vi "To Serial Form.vi"(6 "Serial Version":T1, 10 "Serializer in":refnum<class "Serializer.lvclass">, 11 "PAS Data in":refnum<class "PAS Data.lvclass">) -> (0 "error out":errorcluster, 2 "Serializer out":refnum<class "Serializer.lvclass">, 3 "PAS Data out":refnum<class "PAS Data.lvclass">)   [LabVIEW 2014, in "PAS Data.lvclass"]
uses:
  PAS Data.lvclass
  <vilib>/NI/AQ Character Lineator/Serializer/Serializer.lvclass
  <vilib>/NI/AQ Character Lineator/Serialization Common/Serial Version.ctl
  PAS Data.lvclass/PAS Data.ctl
  Cell/PAS Cell Data.lvclass
  <vilib>/NI/AQ Character Lineator/Serializable/Insert Boolean.vi
  <vilib>/NI/AQ Character Lineator/Serializer/Insert Boolean.vi
  <vilib>/NI/AQ Character Lineator/Serializer/Read Include Default Values.vi
  Data/Data.lvclass
  <vilib>/NI/AQ Character Lineator/Serializable/Serializable.lvclass
  <vilib>/NI/AQ Character Lineator/Serialization Common/Serialization Common.lvlib
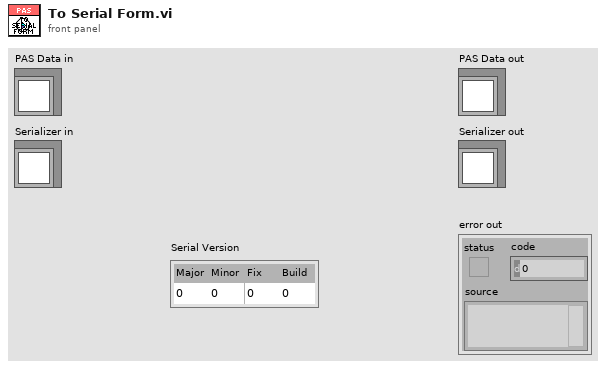
[diagram p1: front panel]
types:
  T1 = typedef "Serialization Common.lvlib/Serial Version.ctl" = cluster{"Major":u16, "Minor":u16, "Fix":u16, "Build":u16}
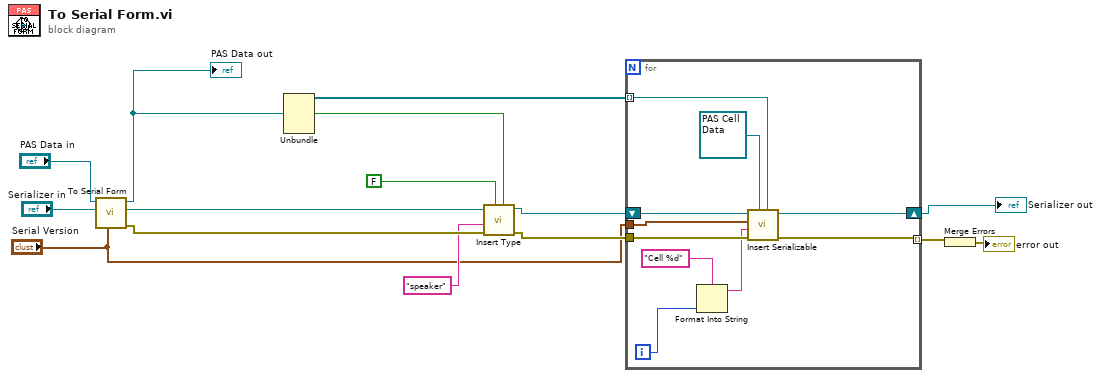
[diagram p0: block diagram]
diagram:
  n1 = call-parent "To Serial Form.vi"("Serial Version"="Serial Version", "Serializer in"="Serializer in", "Data in"="PAS Data in") -> ("error out"=w11:errorcluster, "Serializer out"=w12:refnum<class "Serializer.lvclass">, "Data out"=w13:refnum<class "PAS Data.lvclass">)  [unwired: 6 in]
  "PAS Data out" <- w13
  n2 = Unbundle(w13) -> (w7:refnum<class "PAS Cell Data.lvclass">[], w10:bool)  [unwired: 3 out]
  n3 = call-poly <vilib>:"Insert Type.vi"("Boolean"=w10, "Default Value"=FALSE, "error in (no error)"=w11, "Name"="speaker", "Serializer in"=w12) -> ("error out"=w5:errorcluster, "Serializer out"=w6:refnum<class "Serializer.lvclass">)  [unwired: 5 in]
  n4 = for {
    tunnel: w7 -> [w25] mode=indexing
    shift-right: [w22] -> w3
    shift-left: w6 -> [w23]
    tunnel: w5 -> [w21]
    tunnel: "Serial Version" -> [w17]
    tunnel: [w16] -> w1 mode=indexing
    i -> [w20]
    n5 = Format Into String(format string="Cell %d", w20) -> (resulting string=w18:string)  [unwired: 2 in, 1 out]
    n6 = call <vilib>:"Insert Serializable.vi"("Serializable"=w25, "Default Value"=refnum<class "PAS Cell Data.lvclass"> refnum ("Cell Data"), "error in (no error)"=w21, "Name"=w18, "Serial Version"=w17, "Serializer in"=w23) -> ("error out"=w16:errorcluster, "Serializer out"=w22:refnum<class "Serializer.lvclass">)  [unwired: 4 in]
  }
  "Serializer out" <- w3
  n7 = Merge Errors(w1) -> (→"error out":errorcluster)
